vi "JSON to Table (SubVI).vi"(8 "error in":errorcluster, 10 "JSON":string, 11 "$Path or Item Name":string) -> (0 "error out":errorcluster, 3 "Array":string[][](array[string]))   [LabVIEW 2017, in "LV_Unicorn.lvlib"]
uses:
  LV_Unicorn.lvlib
  <vilib>/JDP Science/JSONtext/JSONtext.lvlib
panel:
  out "Item Names":string[](array[string])
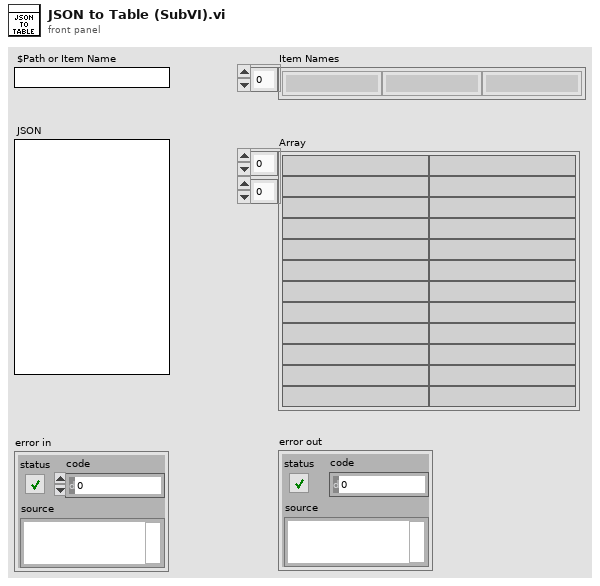
[diagram p1: front panel]
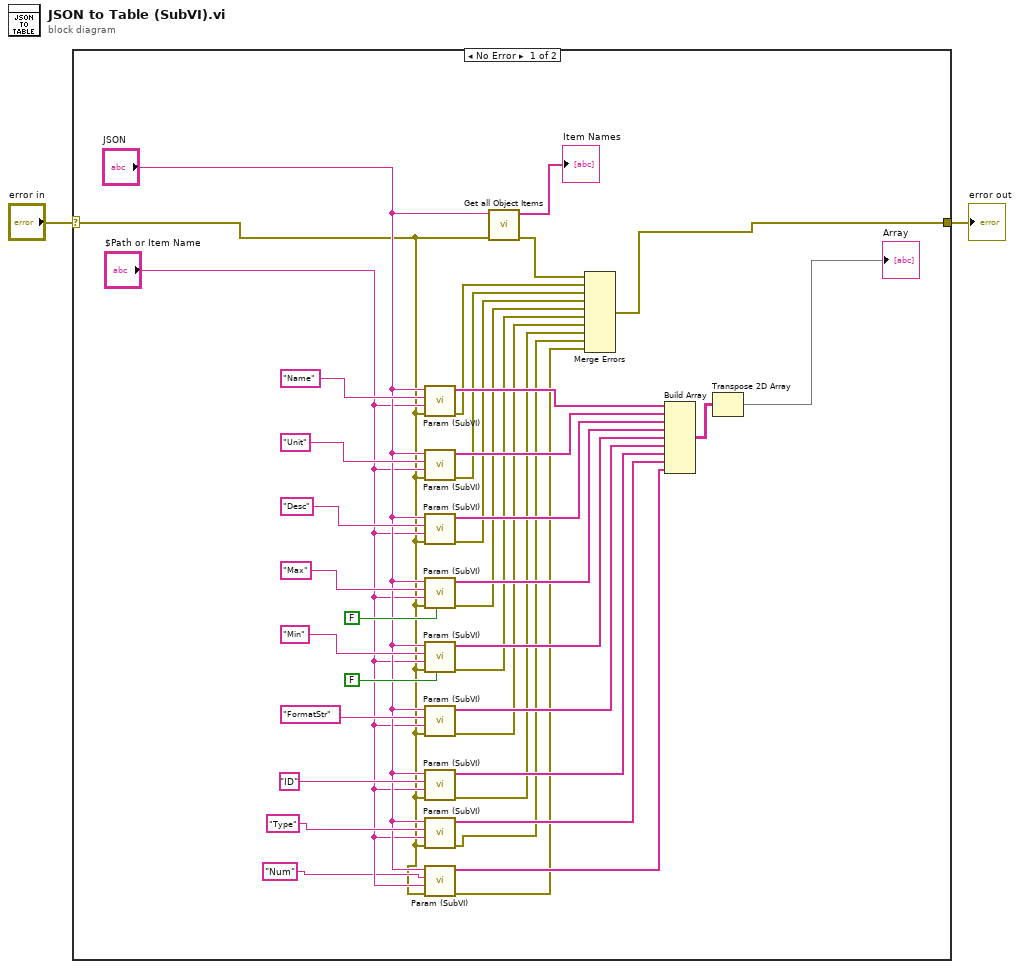
[diagram p0: block diagram]
diagram:
  n1 = case shown="No Error" "error in" {
    selector: "error in" -> [w6 w40]
    tunnel: [w12 w40] -> w2
    frame No Error {
      n2 = call "Param (SubVI).vi"("error in"=w6, "Item"="$Path or Item Name", "Param"="Name" ("$Path or Item Name"), "<JSON>"="JSON") -> ("error out"=w20:errorcluster, "Array"=w29:string[])  [unwired: 6 in]
      n3 = call "Param (SubVI).vi"("error in"=w6, "Item"="$Path or Item Name", "Param"="Unit" ("$Path or Item Name"), "<JSON>"="JSON") -> ("error out"=w19:errorcluster, "Array"=w30:string[])  [unwired: 6 in]
      n4 = call "Param (SubVI).vi"("error in"=w6, "Item"="$Path or Item Name", "Param"="Desc" ("$Path or Item Name"), "<JSON>"="JSON") -> ("error out"=w18:errorcluster, "Array"=w31:string[])  [unwired: 6 in]
      n5 = call "Param (SubVI).vi"("Удалить кавычки"=FALSE, "error in"=w6, "Item"="$Path or Item Name", "Param"="Max" ("$Path or Item Name"), "<JSON>"="JSON") -> ("error out"=w17:errorcluster, "Array"=w36:string[])  [unwired: 5 in]
      n6 = call "Param (SubVI).vi"("Удалить кавычки"=FALSE, "error in"=w6, "Item"="$Path or Item Name", "Param"="Min" ("$Path or Item Name"), "<JSON>"="JSON") -> ("error out"=w16:errorcluster, "Array"=w37:string[])  [unwired: 5 in]
      n7 = call "Param (SubVI).vi"("error in"=w6, "Item"="$Path or Item Name", "Param"="FormatStr" ("$Path or Item Name"), "<JSON>"="JSON") -> ("error out"=w15:errorcluster, "Array"=w39:string[])  [unwired: 6 in]
      n8 = call "Param (SubVI).vi"("error in"=w6, "Item"="$Path or Item Name", "Param"="ID" ("$Path or Item Name"), "<JSON>"="JSON") -> ("error out"=w14:errorcluster, "Array"=w24:string[])  [unwired: 6 in]
      n9 = call "Param (SubVI).vi"("error in"=w6, "Item"="$Path or Item Name", "Param"="Type" ("$Path or Item Name"), "<JSON>"="JSON") -> ("error out"=w4:errorcluster, "Array"=w10:string[])  [unwired: 6 in]
      n10 = call "Param (SubVI).vi"("error in"=w6, "Item"="$Path or Item Name", "Param"="Num" ("$Path or Item Name"), "<JSON>"="JSON") -> ("error out"=w3:errorcluster, "Array"=w5:string[])  [unwired: 6 in]
      n11 = call <vilib>:"Get all Object Items.vi"("error in (no error)"=w6, "JSON"="JSON") -> ("error out"=w13:errorcluster, "Item Names"=→"Item Names":string[])  [unwired: 6 in, 2 out]
      n12 = Merge Errors(w13, w20, w19, w18, w17, w16, w15, w14, w4, w3) -> (w12:errorcluster)
      n13 = Build Array(w29, w30, w31, w36, w37, w39, w24, w10, w5) -> (w32:string[][])
      n14 = Transpose 2D Array(2D array=w32) -> (transposed array=→"Array":string[][])
    }
    frame Error {
    }
  }
  "error out" <- w2
